vi "XML_Get Tag.vi"(8 "error in (no error)":errorcluster, 10 "Tag name":string, 11 "XML String in":string) -> (0 "error out":errorcluster, 1 "Remaining string":string, 2 "Tag value":string, 3 "XML String dup":string, 5 "Tag attributes":string)   [LabVIEW 2015, in "XML Parser.lvlib"]
uses:
  XML Parser.lvlib
  <vilib>/regexp/Match Regular Expression.xnode
panel:
  out "Whole tag":string
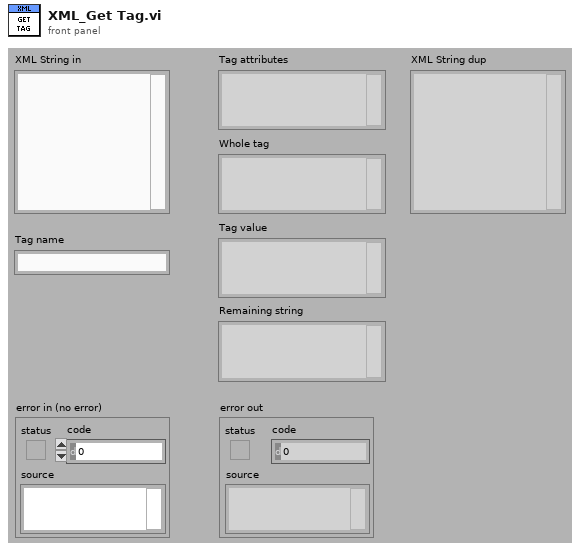
[diagram p1: front panel]
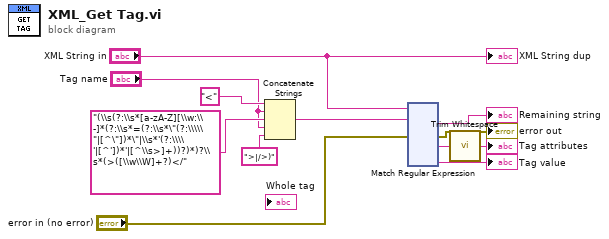
[diagram p0: block diagram]
diagram:
  n1 = Concatenate Strings("<", "Tag name", "(\\s(?:\\s*[a-zA-Z][\\w:\\-]*(?:\\s*=(?:\\s*\"(?:\\\\\"|[^\"])*\"|\\s*'(?:\\\\'|[^'])*'|[^\\s>]+))?)*)?\\s*(>([\\w\\W]+?)</", "Tag name", ">|/>)" ("string")) -> (w8:string)
  n2 = xnode "Match Regular Expression"("input string"="XML String in", "regular expression"=w8, "error in"="error in (no error)") -> ("after match"=→"Remaining string":string, "error out"=→"error out":errorcluster, "submatch 1"=w3:string, "submatch 3"=→"Tag value":string)  [unwired: 3 in, 4 out]
  n3 = call <vilib>:"Trim Whitespace.vi"("string"=w3) -> ("trimmed string"=→"Tag attributes":string)  [unwired: 1 in]
  "XML String dup" <- "XML String in"
